vi "tvac_gui_v3.vi"() -> ()   [LabVIEW 2017]
uses:
  <vilib>/httpClient/ClientHandle.ctl
  msg7171_linux.llb/send single message.vi
  <vilib>/httpClient/POSTBuffer.vi
  <vilib>/httpClient/LabVIEWHTTPClient.lvlib
panel:
  in  "NumberTCs":i32=10
  out "Plot.Plot Color":u32
  in  "alarm":i32
  out "String 2":string
  in  "Tab Control":enum32{"Page 1", "Page 2"}(tab)
  in  "Zone 1":T1 {"Ring" items=["Average", "Maximum", "Minimum", ""]}
  out "thermocouple":T2(array[cluster]) {"Numeric" format="%#.2g"}
  out "Waveform Chart":waveform(dbl)[](graph)
  in  "exit":bool
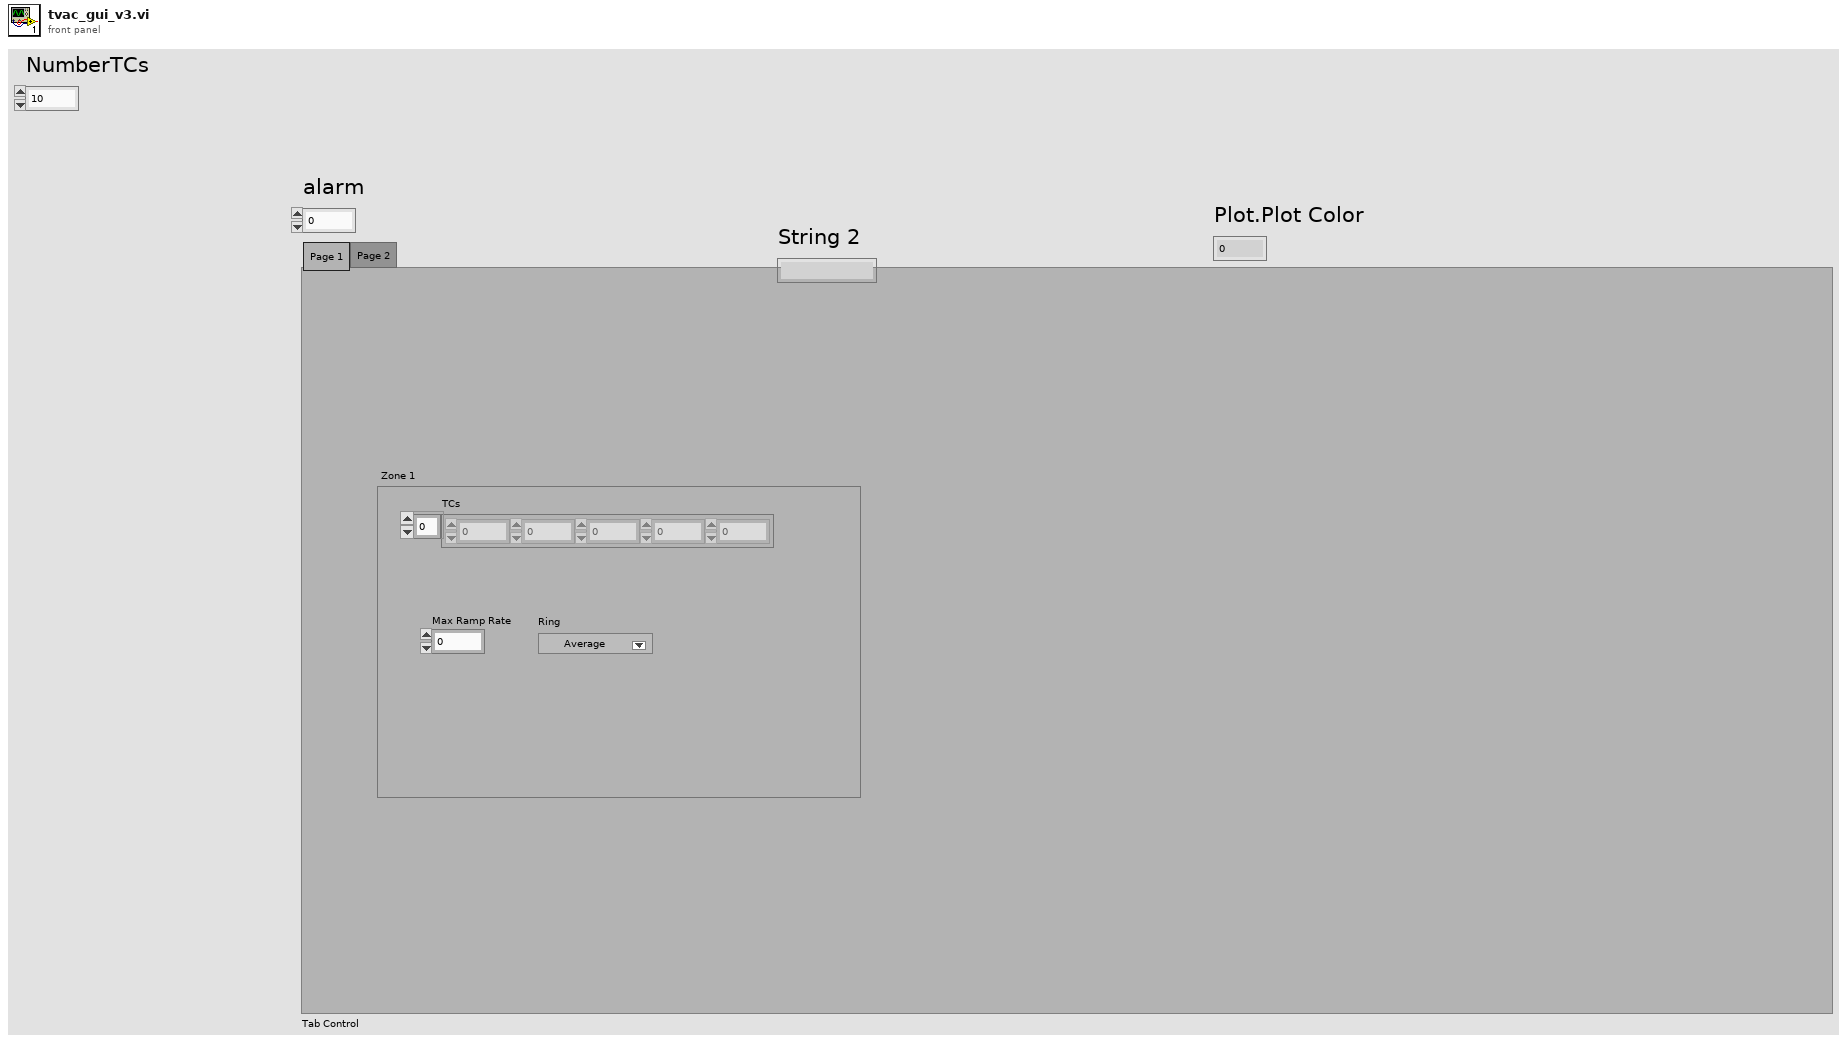
[diagram p1: front panel]
types:
  T1 = cluster{"Ring":u16, "Max Ramp Rate":dbl, "TCs":dbl[]}
  T2 = cluster{"Numeric":dbl, "Color Box":u32, "String":string, "PlotColor":u32}[][]
  T3 = typedef "LabVIEWHTTPClient.lvlib/ClientHandle.ctl" = refnum<k1>
  T4 = cluster{"go":bool, "Http session":T3, "URL prefex":string}
  T5 = typedef "LVPoint32TypeDef.ctl" = cluster{"Horizontal":i32, "Vertical":i32}
  T6 = typedef "LVPositionTypeDef.ctl" = cluster{"Left":i32, "Top":i32}
  T7 = cluster{"Numeric":dbl, "Color Box":u32, "String":string, "PlotColor":u32}
  T8 = cluster{"time":string, "tcs":cluster{"thermocouple":i32, "time":i32, "temp":i32, "working":i32, "alarm":i32}[]}
  T9 = cluster{"thermocouple":i32, "time":i32, "temp":i32, "working":i32, "alarm":i32}[]
  T10 = cluster{"thermocouple":i32, "time":i32, "temp":i32, "working":i32, "alarm":i32}
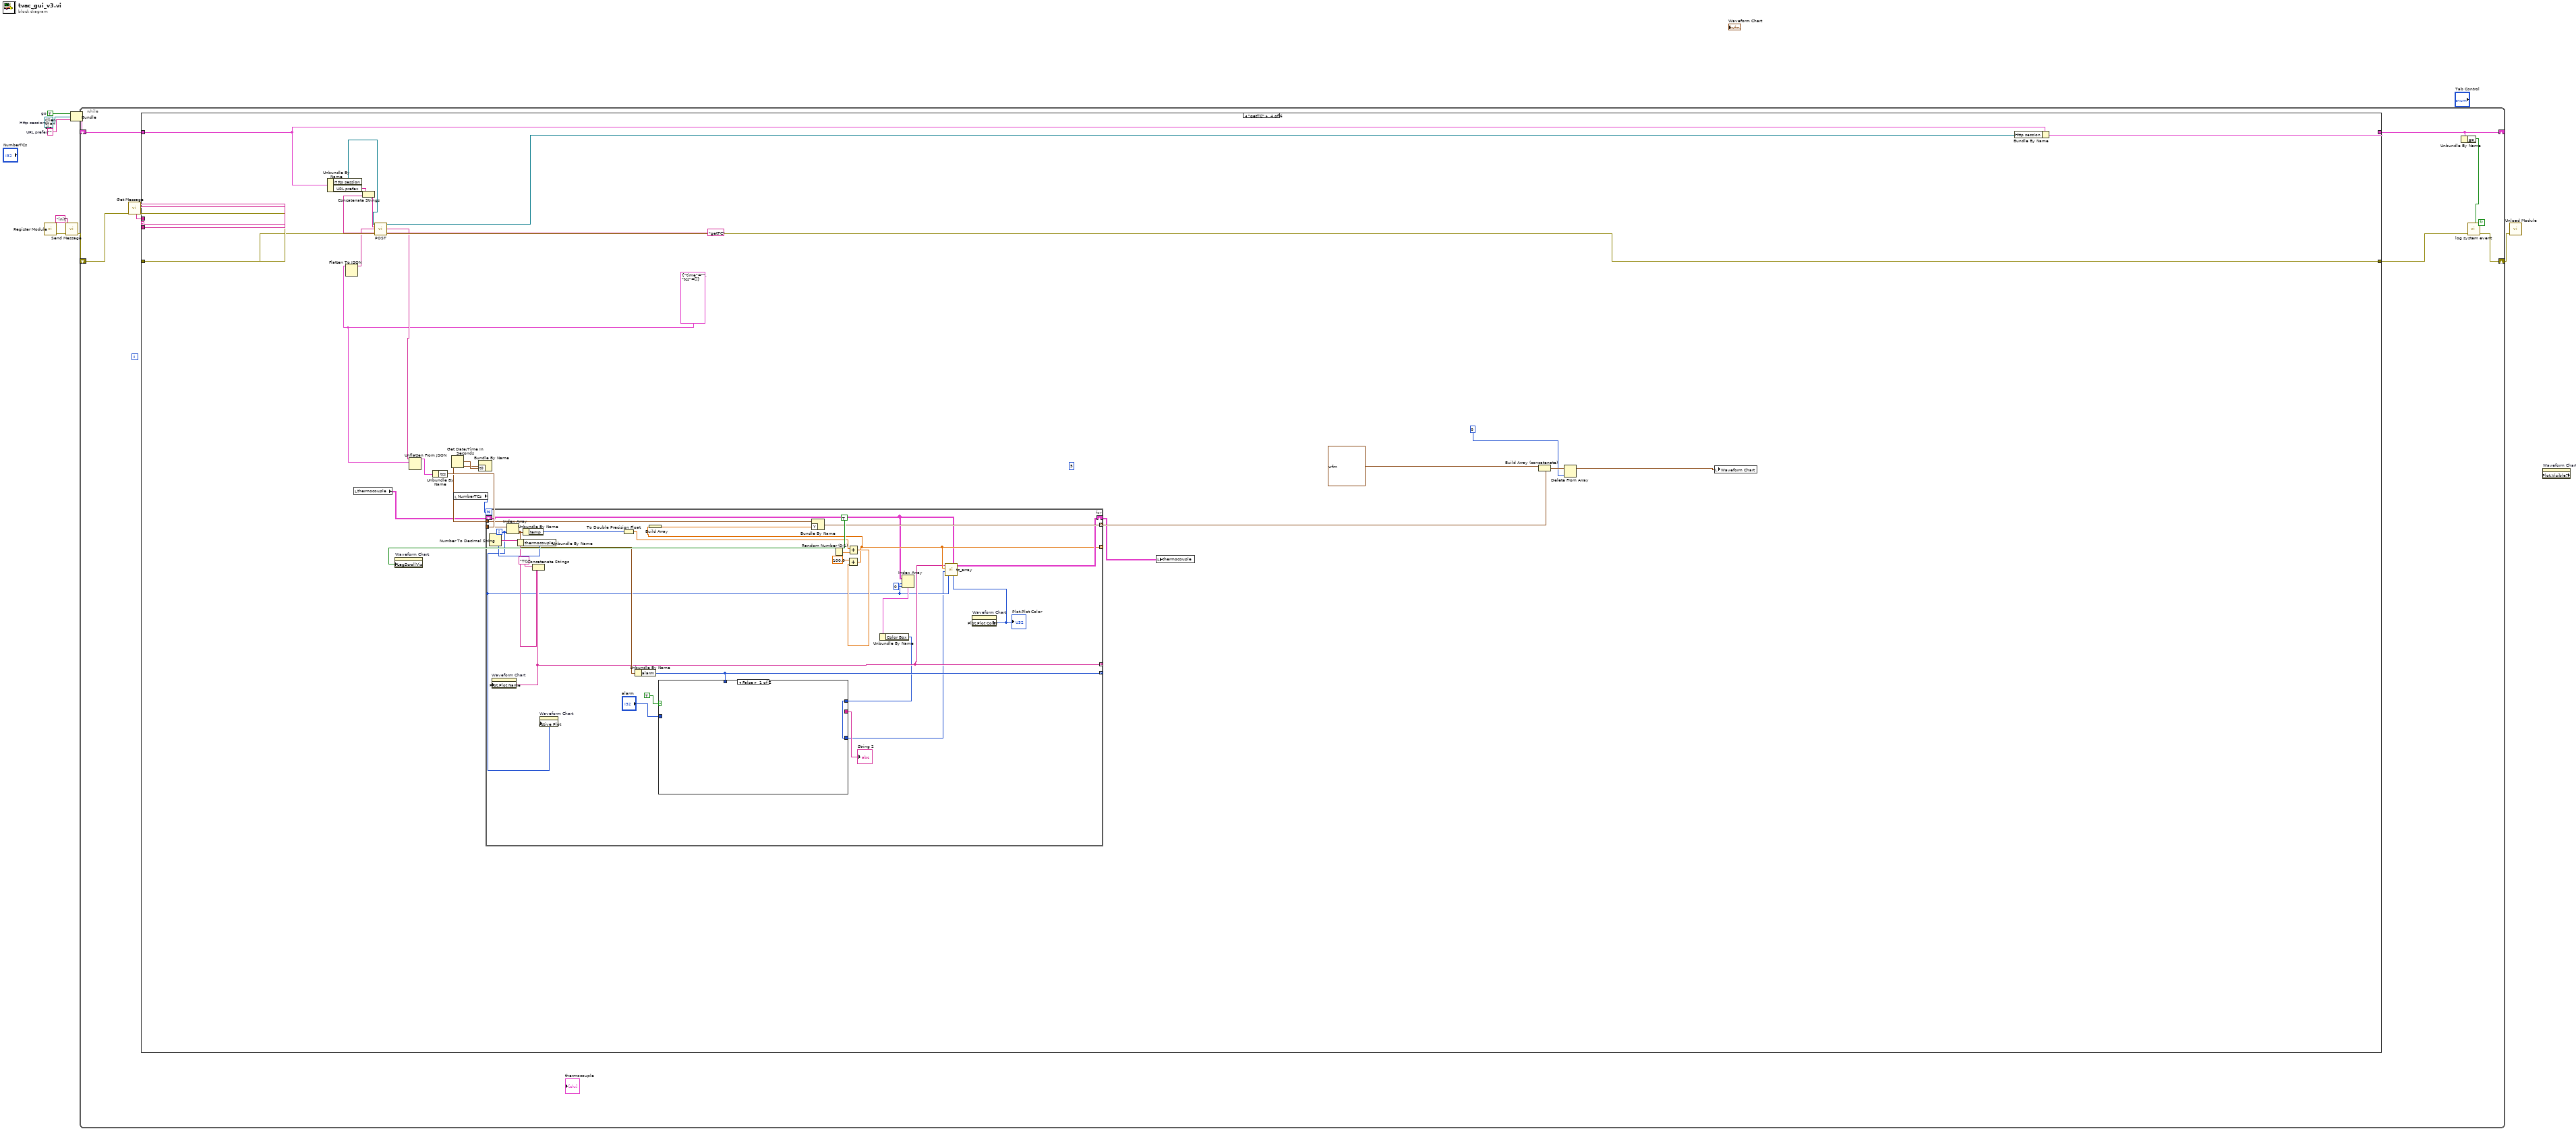
[diagram p0: block diagram]
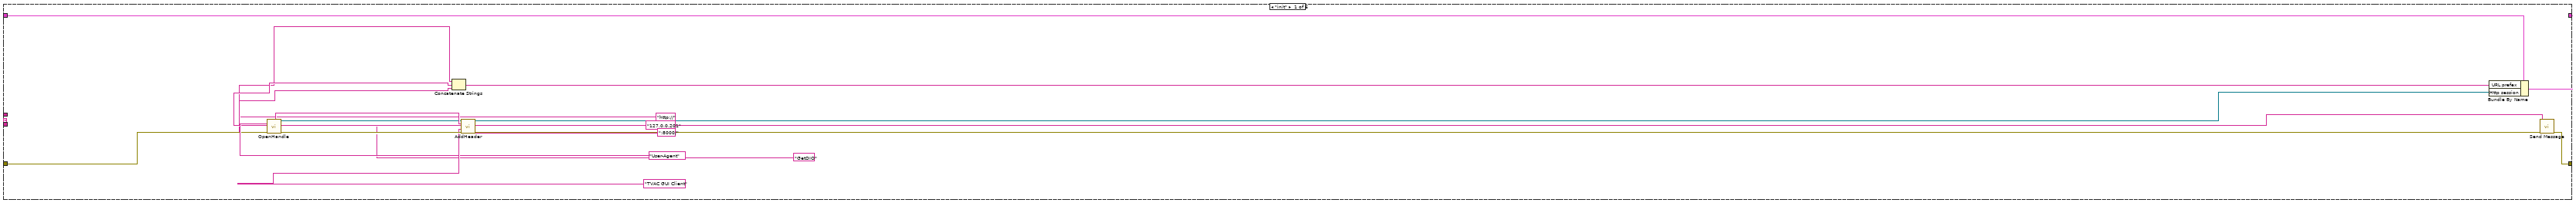
[diagram p2: hidden frame]
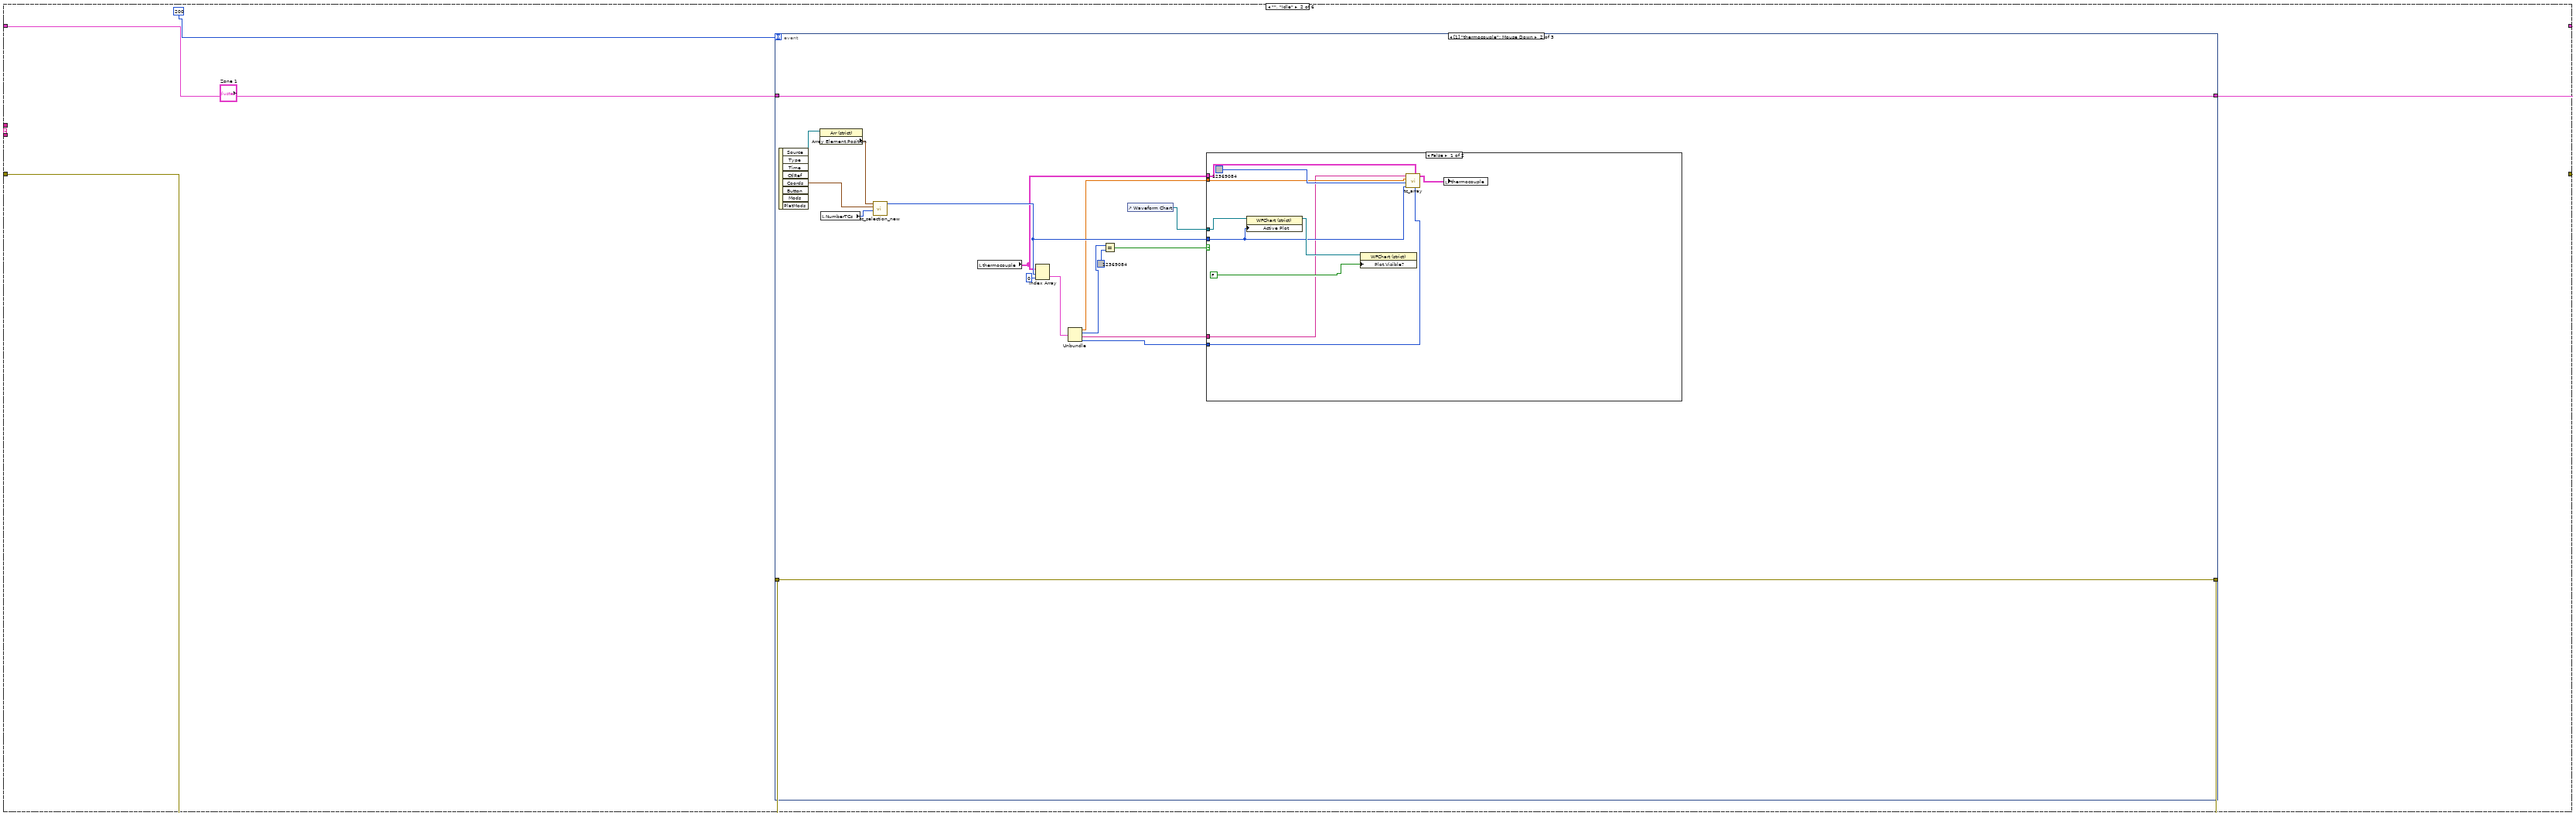
[diagram p3: hidden frame]
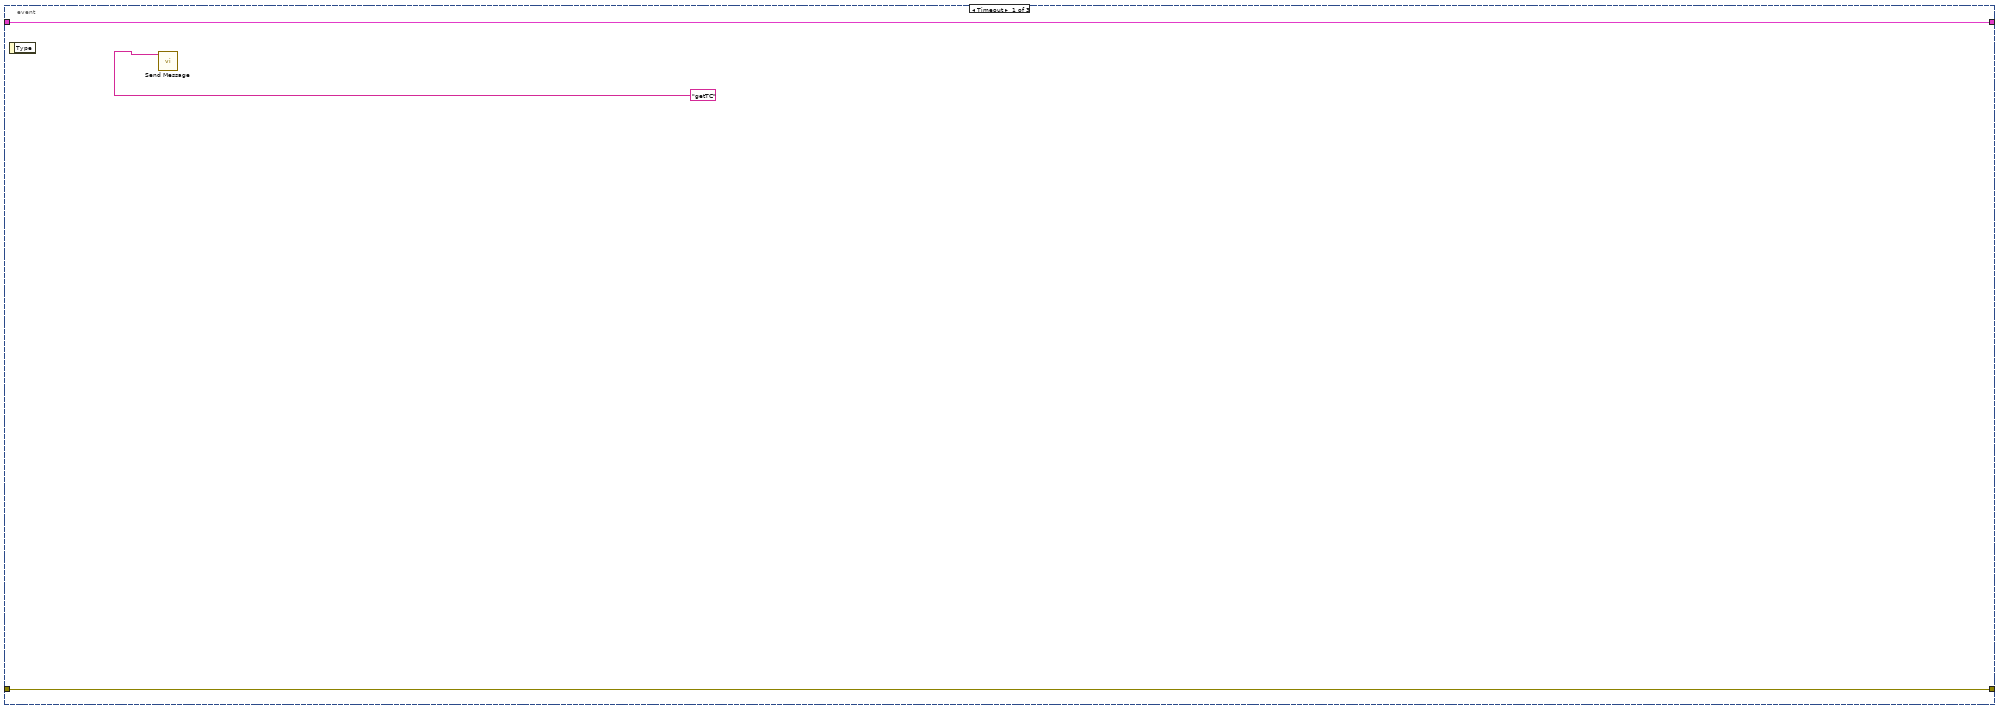
[diagram p4: hidden frame]
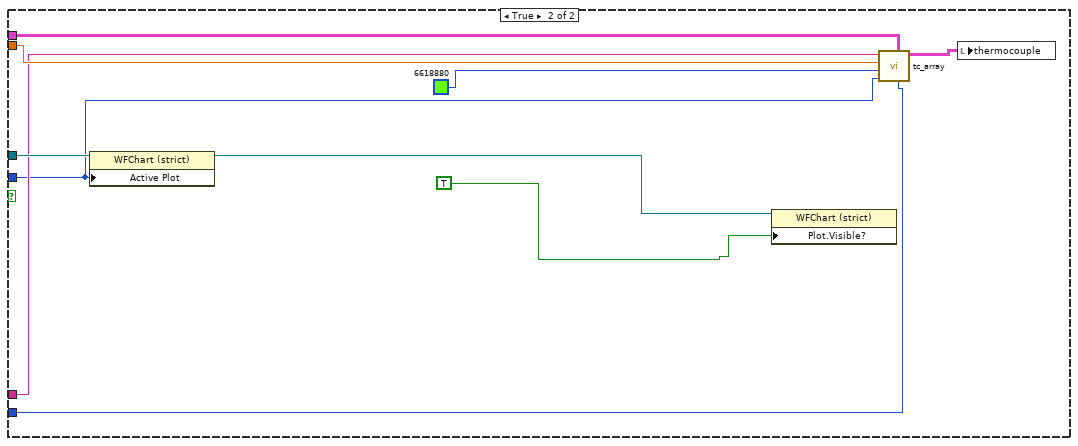
[diagram p5: hidden frame]
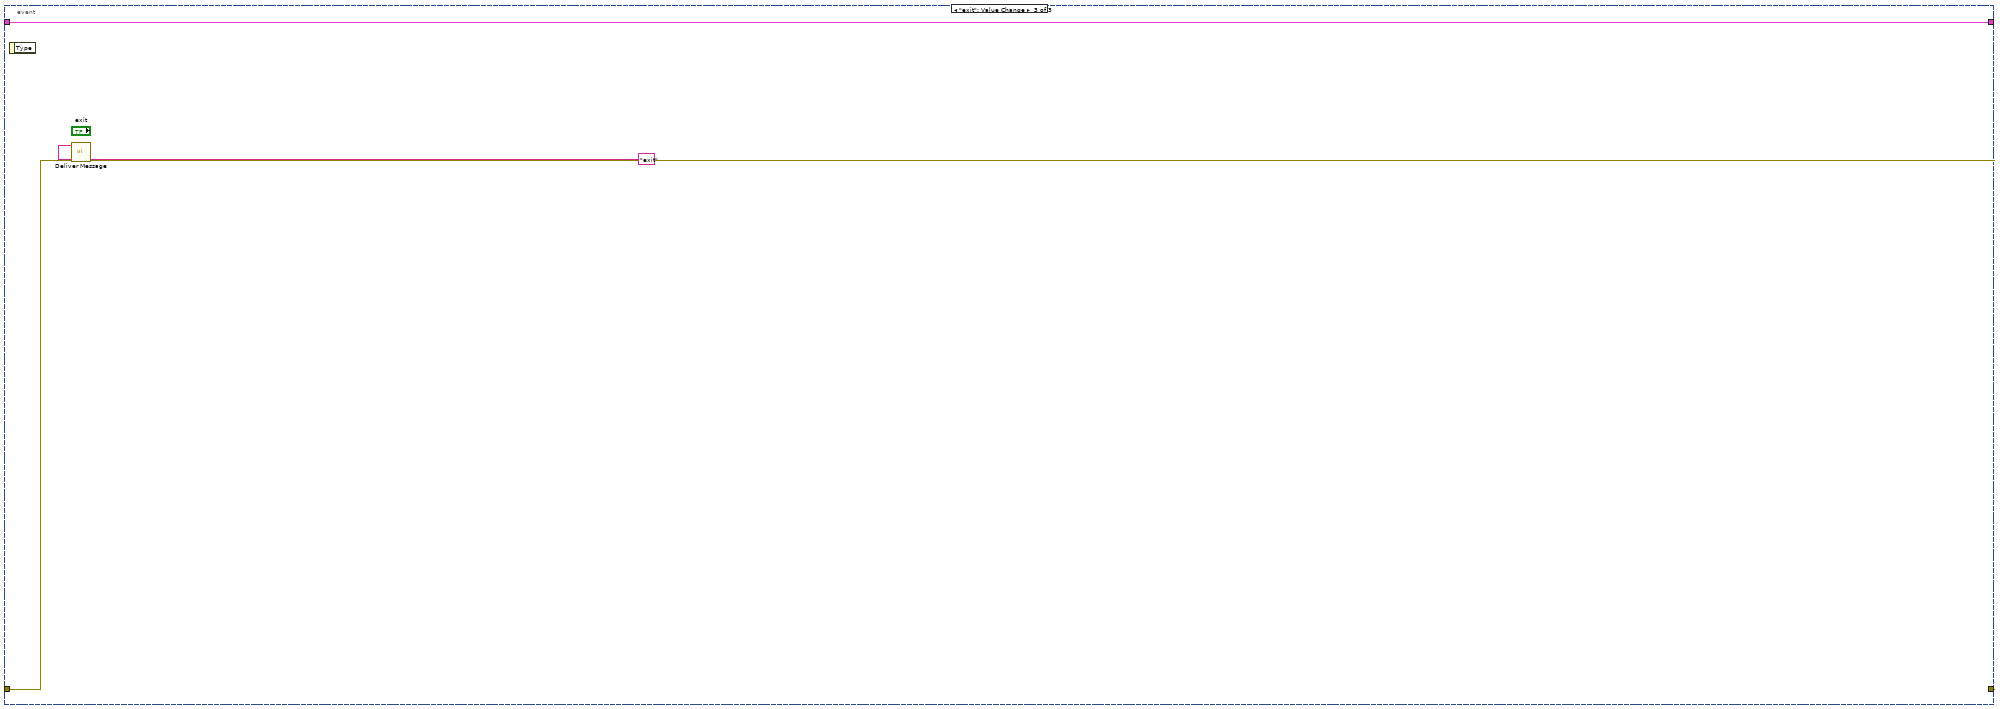
[diagram p6: hidden frame]
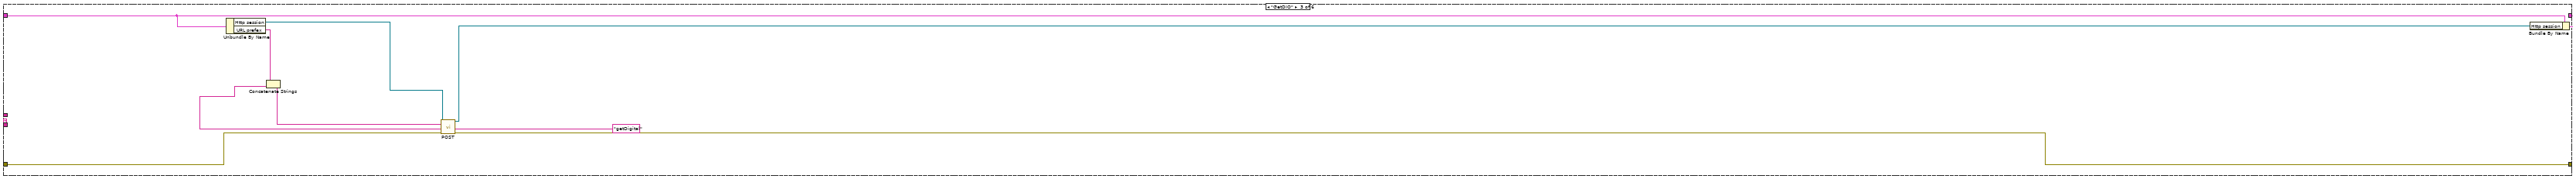
[diagram p7: hidden frame]
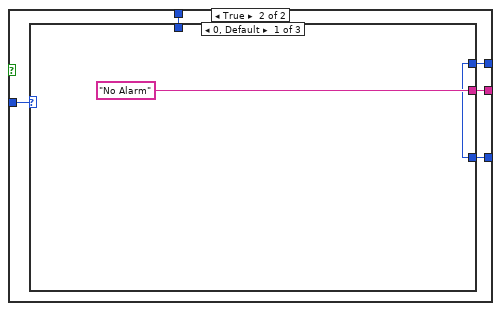
[diagram p8: hidden frame]
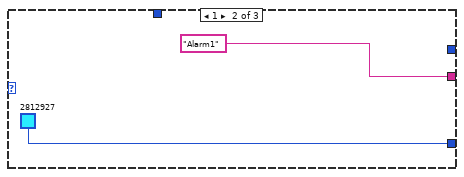
[diagram p9: hidden frame]
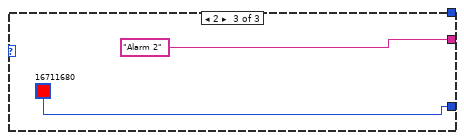
[diagram p10: hidden frame]
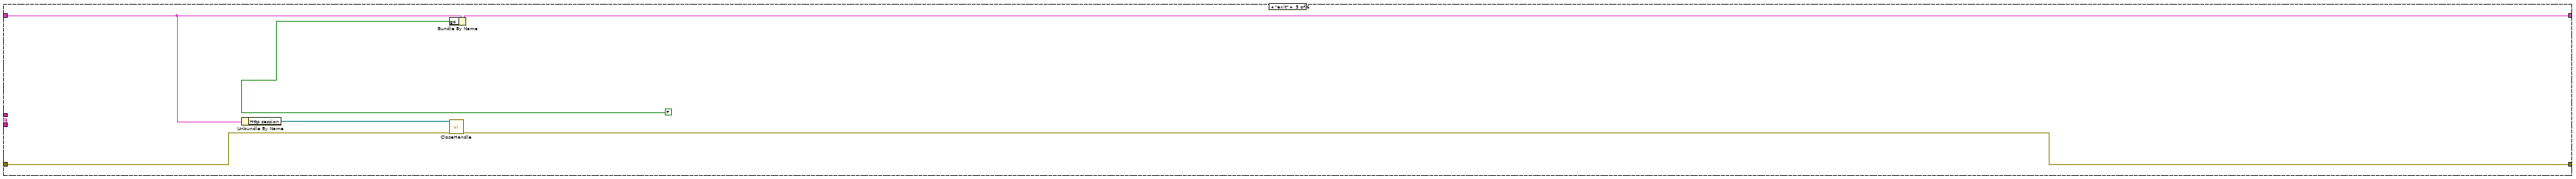
[diagram p11: hidden frame]
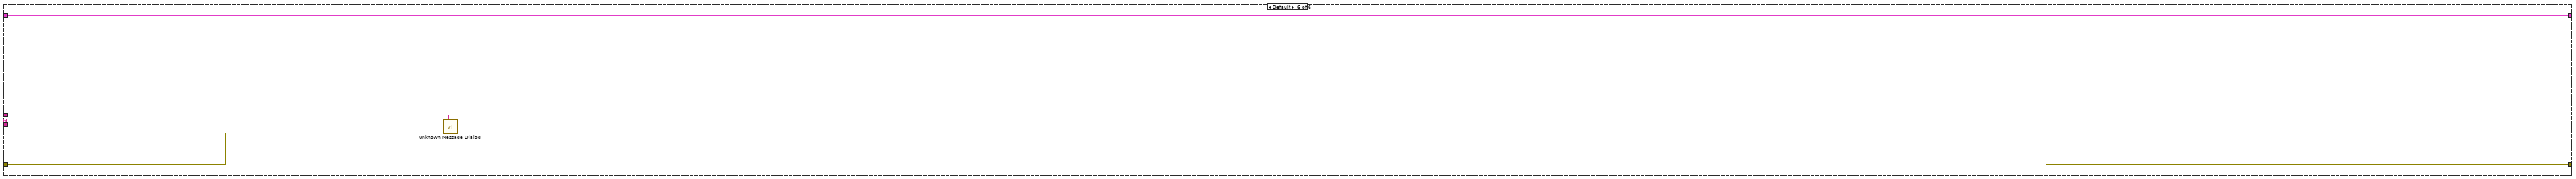
[diagram p12: hidden frame]
diagram:
  w4 = ""  # URL prefex
  w5 = T3 refnum  # Http session
  w6 = TRUE  # go
  n1 = call "Register Module.vi"() -> ("error out"=w2:errorcluster)  [unwired: 10 in, 1 out]
  n2 = call-poly "Send Message.vi"("error in (no error)"=w2, "event"="init") -> ("error out"=w1:errorcluster)  [unwired: 9 in]
  n3 = Bundle("go"=w6, "Http session"=w5, "URL prefex"=w4) -> (w8:T4)  [unwired: 1 in]
  n4 = while {
    shift-left: w8 -> [w15]
    shift-right: [w12] -> _
    shift-right: [w10] -> w7
    shift-left: w1 -> [w18]
    stop <- w11 continue-if-true
    n5 = call "Get Message.vi"("error in (no error)"=w18) -> ("error out"=w16:errorcluster, "event buffer"=w17:string, "event"=w14:string, "source"=w13:string)  [unwired: 7 in]
    n6 = case shown="\"getTC\"" w14 {
      selector: w14 -> [_ _ _ _ _ w164]
      tunnel: [w24 w35 w84 w114 w161 w166] -> w12
      tunnel: w15 -> [w33 w34 w83 w112 w156 w166]
      tunnel: w17 -> [_ _ _ _ _ _]
      tunnel: w16 -> [w28 w36 w86 w116 w159 w165]
      tunnel: w13 -> [_ _ _ _ _ w163]
      tunnel: [w20 w38 w85 w115 w158 w162] -> w9
      frame "init" {
        n7 = call <vilib>:"OpenHandle.vi"("error in (no error)"=w28) -> ("client handle out"=w29:T3, "error out"=w32:errorcluster)  [unwired: 13 in]
        n8 = Concatenate Strings("http://" ("url"), "127.0.0.201" ("Address"), ":8000/" ("url")) -> (w23:string)
        n9 = call <vilib>:"AddHeader.vi"("client handle"=w29, "header"="User-Agent", "value"="TVAC GUI Client", "error in (no error)"=w32) -> ("client handle out"=w22:T3, "error out"=w21:errorcluster)  [unwired: 10 in]
        n10 = Bundle By Name(cluster=w33, "URL prefex"=w23, "Http session"=w22) -> (w24:T4)
        n11 = call-poly "Send Message.vi"("error in (no error)"=w21, "event"="GetDIO") -> ("error out"=w20:errorcluster)  [unwired: 9 in]
      }
      frame "", "Idle" {
        n12 = event shown="[1] \"thermocouple\": Mouse Down" {
          selector: _ -> [_ _ _]
          dyn-events: _ -> [_ _ _]
          timeout: 200 ("milliseconds to wait") -> [_ _ _]
          tunnel: w36 -> [w40 w58 w82]
          tunnel: [w40 w58 w81] -> w38
          tunnel: [w41 w57 w79] -> w35
          tunnel: w34 -> [w41 w57 w79]
          event Timeout {
            n13 = event-data() -> ()  [unwired: 1 in, 1 out]
            n14 = call-poly "Send Message.vi"("event"="getTC") -> ()  [unwired: 10 in, 1 out]
          }
          event "thermocouple": Mouse Down {
            n15 = event-data() -> ("CtlRef"=w54:refnum<vi>, "Coords"=w55:T5)  [unwired: 1 in, 6 out]
            n16 = property class="Arr (strict)"(reference=w54) -> ("Array Element.Position"=w56:T6)  [unwired: 1 in, 2 out]
            n17 = local read "NumberTCs"() -> (w42:i32)
            n18 = call "tc_selection_new.vi"("Numeric 2"=w42, "Coords"=w55, "Position"=w56) -> ("Numeric"=w48:i32)  [unwired: 8 in]
            n19 = local read "thermocouple"() -> (w46:T2)
            n20 = Index Array(array=w46, index (row)=w48, index (col)=0 ("disabled index (col)")) -> (element=w51:T7)
            n21 = Unbundle(w51) -> ("Numeric"=w45:dbl, "Color Box"=w50:u32, "String"=w44:string, "PlotColor"=w43:u32)
            n22 = Equal?(x=w50, y=u32 12369084) -> (x = y?=w49:bool)
            n23 = control-ref of="Waveform Chart"() -> (w47:refnum<vi>)
            n24 = case shown="False" w49 {
              tunnel: w48 -> [w65 w73]
              tunnel: w47 -> [w66 w76]
              tunnel: w46 -> [w59 w70]
              tunnel: w45 -> [w63 w75]
              tunnel: w44 -> [w62 w74]
              tunnel: w43 -> [w60 w71]
              frame False {
                n25 = property on="Property Node" class="WFChart (strict)"(reference=w66, "Active Plot"=w65) -> (reference out=w67:refnum<vi>)  [unwired: 1 in, 1 out]
                n26 = property class="WFChart (strict)"(reference=w67, "Plot.Visible?"=FALSE ("Plot.Visible")) -> ()  [unwired: 1 in, 2 out]
                n27 = call "tc_array.vi"("String"=w62, "Numeric"=w63, "Color Box"=u32 12369084, "index (row)"=w65, "output array 2"=w59, "PlotColor"=w60) -> ("output array"=w61:T2)  [unwired: 3 in]
                n28 = local write "thermocouple"(w61) -> ()
              }
              frame True {
                n29 = property class="WFChart (strict)"(reference=w76, "Active Plot"=w73) -> (reference out=w77:refnum<vi>)  [unwired: 1 in, 1 out]
                n30 = property class="WFChart (strict)"(reference=w77, "Plot.Visible?"=TRUE ("Plot.Visible")) -> ()  [unwired: 1 in, 2 out]
                n31 = call "tc_array.vi"("String"=w74, "Numeric"=w75, "Color Box"=u32 6618880, "index (row)"=w73, "output array 2"=w70, "PlotColor"=w71) -> ("output array"=w69:T2)  [unwired: 3 in]
                n32 = local write "thermocouple"(w69) -> ()
              }
            }
          }
          event "exit": Value Change {
            n33 = event-data() -> ()  [unwired: 1 in, 1 out]
            n34 = call "Deliver Message.vi"("error in (no error)"=w82, "event"="exit") -> ("error out"=w81:errorcluster)  [unwired: 9 in]
          }
        }
      }
      frame "GetDIO" {
        n35 = Unbundle By Name(w83) -> ("Http session"=w90:T3, "URL prefex"=w88:string)
        n36 = Concatenate Strings(w88, "getDigital" ("url")) -> (w89:string)
        n37 = call-poly <vilib>:"POST.vi"("client handle"=w90, "url"=w89, "error in (no error)"=w86) -> ("client handle out"=w91:T3, "error out"=w85:errorcluster)  [unwired: 9 in, 2 out]
        n38 = Bundle By Name(cluster=w83, "Http session"=w91) -> (w84:T4)
      }
      frame "getTC" {
        (unwired) 5
        w105 = T8 {"time"="", "tcs"=[]}
        n39 = Unbundle By Name(w112) -> ("Http session"=w111:T3, "URL prefex"=w109:string)
        n40 = Flatten To JSON(anything=w105) -> (JSON string=w107:string)  [unwired: 2 in, 1 out]
        n41 = local read "thermocouple"() -> (w95:T2)
        n42 = Concatenate Strings(w109, "getTC" ("url")) -> (w110:string)
        n43 = call-poly <vilib>:"POST.vi"("client handle"=w111, "url"=w110, "buffer"=w107, "error in (no error)"=w116) -> ("client handle out"=w113:T3, "body"=w106:string, "error out"=w115:errorcluster)  [unwired: 8 in, 1 out]
        n44 = property on="Waveform Chart" class="WFChart (strict)"("LegScrollVis"=TRUE ("Legend:Scrollbar Visible")) -> ()  [unwired: 2 in, 2 out]
        n45 = Unflatten From JSON(JSON string=w106, type and defaults=w105) -> (value=w104:T8)  [unwired: 5 in, 1 out]
        n46 = Unbundle By Name(w104) -> ("tcs"=w103:T9)
        n47 = Get Date/Time In Seconds() -> (seconds since 1Jan1904=w100:timestamp)
        n48 = local read "NumberTCs"() -> (w92:i32)
        n49 = Bundle By Name("t0"=w100) -> (w99:waveform(dbl))  [unwired: 1 in]
        n50 = for {
          N: w92 -> [_]
          tunnel: w103 -> [w143]
          tunnel: w99 -> [w141]
          tunnel: [w142] -> w98 mode=indexing
          tunnel: [w123] -> _ mode=indexing
          tunnel: [w122] -> _ mode=indexing
          tunnel: [w125] -> _ mode=indexing
          shift-right: [w124] -> w96
          shift-left: w95 -> [w121]
          i -> [w120]
          n51 = Index Array(array=w143, index=w120) -> (element=w133:T10)
          n52 = Unbundle By Name(w133) -> ("thermocouple"=w139:i32)
          n53 = Number To Decimal String(number=w139) -> (decimal integer string=w140:string)  [unwired: 1 in]
          n54 = Unbundle By Name(w133) -> ("temp"=w137:i32)
          n55 = Concatenate Strings("TC " ("string"), w140) -> (w122:string)
          n56 = property on="Waveform Chart" class="WFChart (strict)"("Plot.Plot Name"=w122) -> ()  [unwired: 2 in, 2 out]
          n57 = property on="Waveform Chart" class="WFChart (strict)"("Active Plot"=w120) -> ()  [unwired: 2 in, 2 out]
          n58 = To Double Precision Float(number=w137) -> (double precision float=w134:dbl)
          n59 = Unbundle By Name(w133) -> ("alarm"=w125:i32)
          n60 = Random Number (0-1)() -> (number: 0 to 1=w135:dbl)
          n61 = Add(x=w134, y=w135) -> (x+y=w131:dbl)
          n62 = Add(x=100.0, y=w131) -> (x+y=w123:dbl)
          n63 = Build Array(w123) -> (w136:dbl[])
          n64 = Bundle By Name(cluster=w141, "Y"=w136) -> (w142:waveform(dbl))
          n65 = Index Array(array=w121, index (row)=w120, index (col)=0 ("disabled index (col)")) -> (element=w128:T7)
          n66 = Unbundle By Name(w128) -> ("Color Box"=w117:u32)
          n67 = case shown="False" TRUE {
            tunnel: [_ w149] -> w130
            tunnel: "alarm" -> [_ w148]
            tunnel: w125 -> [_ w147]
            tunnel: [w144 w146] -> w118
            tunnel: w117 -> [w144 w145]
            frame False {
            }
            frame True {
              n68 = case shown="0, Default" w148 {
                tunnel: ["No Alarm" "Alarm1" "Alarm 2"] -> w149
                tunnel: w147 -> [_ _ _]
                tunnel: [w150 u32 2812927 u32 16711680] -> w146
                tunnel: w145 -> [w150 _ _]
                frame 0, Default {
                }
                frame 1 {
                }
                frame 2 {
                }
              }
            }
          }
          "String 2" <- w130
          n69 = property on="Waveform Chart" class="WFChart (strict)"() -> ("Plot.Plot Color"=w119:u32)  [unwired: 2 in, 2 out]
          "Plot.Plot Color" <- w119
          n70 = call "tc_array.vi"("String"=w122, "Numeric"=w123, "Color Box"=w118, "index (row)"=w120, "output array 2"=w121, "PlotColor"=w119) -> ("output array"=w124:T2)  [unwired: 3 in]
        }
        n71 = local write "thermocouple"(w96) -> ()
        n72 = Build Array (concatenate)(waveform(dbl) {"t0"=timestamp(0 s since 1904-01-01), "dt"=1.0, "Y"=[]} ("element"), w98) -> (w102:waveform(dbl)[])
        n73 = Delete From Array(array=w102, index=0) -> (array with subset deleted=w93:waveform(dbl)[])  [unwired: 1 in, 1 out]
        n74 = local write "Waveform Chart"(w93) -> ()
        n75 = Bundle By Name(cluster=w112, "Http session"=w113) -> (w114:T4)
      }
      frame "exit" {
        n76 = Unbundle By Name(w156) -> ("Http session"=w157:T3)
        n77 = Bundle By Name(cluster=w156, "go"=FALSE ("Bundle Element")) -> (w161:T4)
        n78 = call <vilib>:"CloseHandle.vi"("client handle"=w157, "error in (no error)"=w159) -> ("error out"=w158:errorcluster)  [unwired: 13 in]
      }
      frame Default {
        n79 = call "Unknown Message Dialog.vi"("source"=w163, "error in (no error)"=w165, "event name"=w164) -> ("error out"=w162:errorcluster)  [unwired: 8 in]
      }
    }
    n80 = Unbundle By Name(w12) -> ("go"=w11:bool)
    n81 = call "log system event.vi"("error in (no error)"=w9) -> ("error out"=w10:errorcluster)  [unwired: 9 in, 1 out]
  }
  n82 = call "Unload Module.vi"("error in (no error)"=w7) -> ()  [unwired: 10 in, 1 out]
  n83 = property on="Waveform Chart" class="WFChart (strict)" props=["Plot", "Visible?"]() -> ()  [unwired: 2 in, 3 out]
